vi "Unpack Shortcut Menu Activation.vi"(11 "ShortcutMenuActivationMsg":refnum<class "ShortcutMenuActivationMsg.lvclass">) -> (0 "Coords":T1, 1 "MenuRef":refnum<k9>, 2 "Time":u32, 3 "CtlRef":refnum<vi>, 4 "SubObj":refnum<vi>, 5 "Control Label":string)   [LabVIEW 2017, in "ActorEvents.lvlib" / "ShortcutMenuActivationMsg.lvclass"]
doc: "<License>\nCopyright © 2017 Composed Systems, LLC | All rights reserved\nwww.composed.io\n\nAuthor: Ethan Stern <ethan.stern@composed.io>\n\nThis software is provided \"AS IS\" WITHOUT WARRANTIES, either express or implied, AND IS FOR EDUCATIONAL PURPOSES ONLY.\n</License>"
uses:
  ShortcutMenuActivationMsg.lvclass
  <vilib>/Utility/miscctls.llb/LVPoint32TypeDef.ctl
  ShortcutMenuActivationMsg.lvclass/ShortcutMenuActivationMsg.ctl
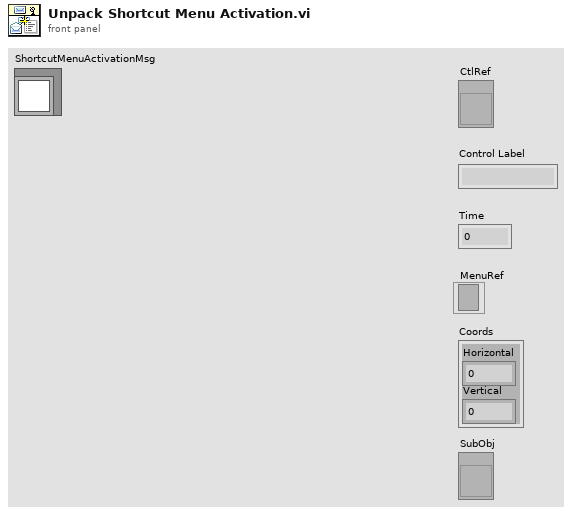
[diagram p1: front panel]
types:
  T1 = typedef "LVPoint32TypeDef.ctl" = cluster{"Horizontal":i32, "Vertical":i32}
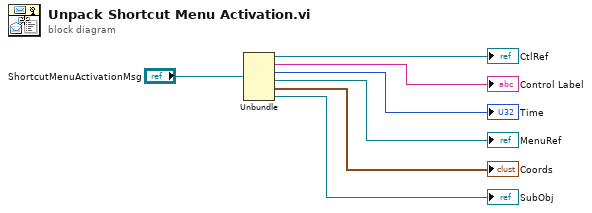
[diagram p0: block diagram]
diagram:
  n1 = Unbundle("ShortcutMenuActivationMsg") -> (→"CtlRef":refnum<vi>, →"Control Label":string, →"Time":u32, →"MenuRef":refnum<k9>, →"Coords":T1, →"SubObj":refnum<vi>)
